vi "unwrap_phase_map.vi"(10 "u8_ar_phase map":u8[][](array[numeric]), 11 "normalize (y)":bool) -> (2 "df_ar_unwrapped_px_ar":dbl[][](array[numeric]), 3 "Refnum out":T1(plugin-control))   [LabVIEW 2011]
doc: "Takes a the warpped phase mapped as a pixel array and unwrappes it. Optional normalization from 0 to 255 for the pixel array output"
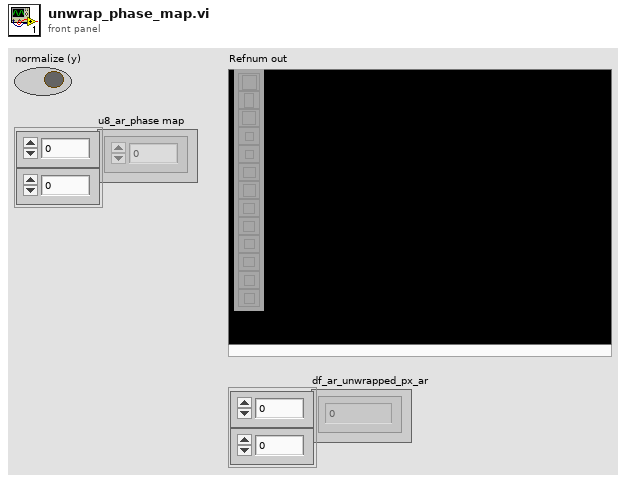
[diagram p1: front panel]
types:
  T1 = typedef "IMAQ Image.ctl" = refnum<image>
  T2 = typedef "Image Type" = u32
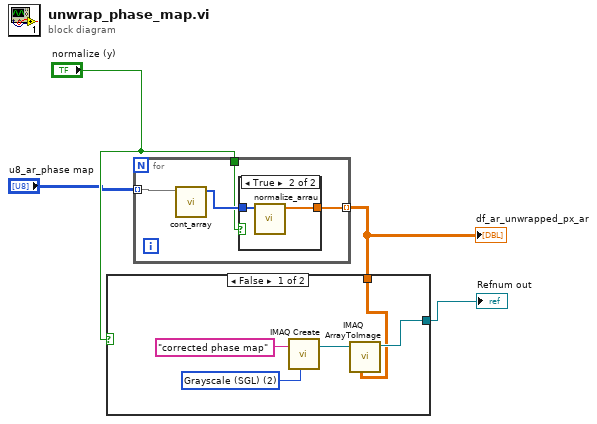
[diagram p0: block diagram]
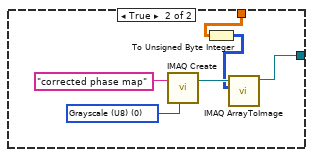
[diagram p2: hidden frame]
diagram:
  n1 = for {
    tunnel: "u8_ar_phase map" -> [w8] mode=indexing
    tunnel: [w6] -> w3 mode=indexing
    tunnel: "normalize (y)" -> [w5]
    n2 = call "cont_array.vi"("u8_ar_phase map"=w8) -> ("Array"=w7:i16[])  [unwired: 10 in]
    n3 = case shown="True" w5 {
      tunnel: w7 -> [w9 w11]
      tunnel: [w9 w10] -> w6
      frame False {
      }
      frame True {
        n4 = call "normalize_arrau.vi"("Array in"=w11) -> ("Array out"=w10:dbl[])  [unwired: 10 in]
      }
    }
  }
  "df_ar_unwrapped_px_ar" <- w3
  n5 = case shown="False" "normalize (y)" {
    tunnel: [w13 w22] -> w2
    tunnel: w3 -> [w12 w18]
    frame False {
      w15 = T2 2 items=["Grayscale (U8)", "Grayscale (I16)", "Grayscale (SGL)", "Complex (CSG)", "RGB (U32)", "HSL (U32)", "RGB (U64)", "Grayscale (U16)"] ("Image Type")
      n6 = call "IMAQ Create"("Image Name"="corrected phase map" ("corrected phase map"), "Image Type"=w15) -> ("New Image"=w16:T1)  [unwired: 2 in, 2 out]
      n7 = call "IMAQ ArrayToImage"("Image Pixels (Float)"=w12, "Image"=w16) -> ("Image Out"=w13:T1)  [unwired: 8 in, 1 out]
    }
    frame True {
      w20 = T2 0 items=["Grayscale (U8)", "Grayscale (I16)", "Grayscale (SGL)", "Complex (CSG)", "RGB (U32)", "HSL (U32)", "RGB (U64)", "Grayscale (U16)"] ("Image Type")
      n8 = call "IMAQ Create"("Image Name"="corrected phase map" ("corrected phase map"), "Image Type"=w20) -> ("New Image"=w21:T1)  [unwired: 2 in, 2 out]
      n9 = To Unsigned Byte Integer(number=w18) -> (unsigned 8bit integer=w17:u8[][])
      n10 = call "IMAQ ArrayToImage"("Image Pixels (U8)"=w17, "Image"=w21) -> ("Image Out"=w22:T1)  [unwired: 8 in, 1 out]
    }
  }
  "Refnum out" <- w2
